vi "SetRessAndName.vi"(8 "error in (no error)":errorcluster caption="entrée d'erreur (pas d'erreur)", 9 "InstrumentName":string, 10 "Nom de ressource VISA":refnum<visa-resource-name>, 11 "BaseDevice en entrée":refnum<class "BaseDevice.lvclass"> caption="DNL_LabVIEW Object in") -> (0 "error out":errorcluster caption="sortie d'erreur", 3 "BaseDevice en sortie":refnum<class "BaseDevice.lvclass"> caption="DNL_LabVIEW Object out")   [LabVIEW 2019, in "BaseDevice.lvclass"]
uses:
  BaseDevice.lvclass
  BaseDevice.lvclass/BaseDevice.ctl
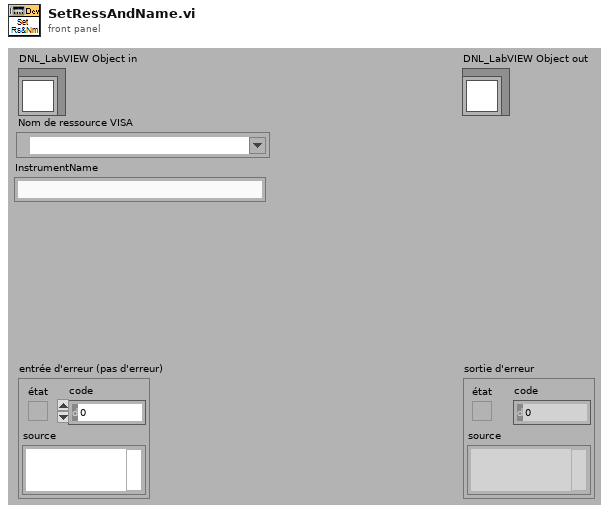
[diagram p1: front panel]
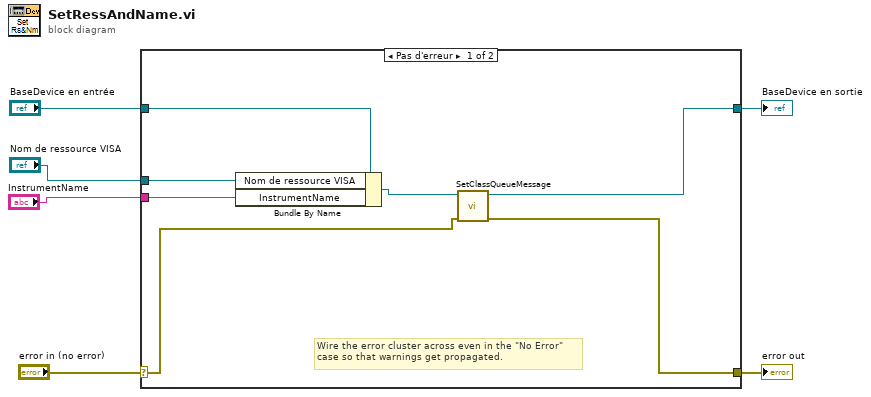
[diagram p0: block diagram]
diagram:
  n1 = case shown="Pas d'erreur" "error in (no error)" {
    selector: "error in (no error)" -> [w8 w15]
    tunnel: [w7 w15] -> w5
    tunnel: [w9 w14] -> w3
    tunnel: "BaseDevice en entrée" -> [w13 w14]
    tunnel: "InstrumentName" -> [w12 _]
    tunnel: "Nom de ressource VISA" -> [w11 _]
    frame No Error {
      # "Wire the error cluster across even in the \"No Error\"\ncase so that warnings get propagated."
      n2 = Bundle By Name(cluster=w13, "Nom de ressource VISA"=w11, "InstrumentName"=w12) -> (w10:refnum<class "BaseDevice.lvclass">)
      n3 = call-dynamic "SetClassQueueMessage.vi"("ErrorIn(No Error)"=w8, "BaseDevice.lvclass"=w10) -> ("sortie d'erreur"=w7:errorcluster, "BaseDevice.lvclass Out"=w9:refnum<class "BaseDevice.lvclass">)  [unwired: 8 in]
    }
    frame Error {
    }
  }
  "error out" <- w5
  "BaseDevice en sortie" <- w3
